vi "Magnet device cluster to String.vi"(11 "Magnet PSU":T1={"Nickname"="", "Bipolar Output"="", "Out Config"="SERS", "Current Limit"=0.0, "AtoB"=0.0, "Inductance"=0.0, "Switch Present"="", "Swh Htr Current"=0.0, "SW VLIM"=0.0, "Ignore Voltage Transient"="", "V Trans Time"=0.0, "Magnet PSU Signals"={"Target Current"=0.0, "Target Field"=0.0, "Target Current Rate"=0.0, "Target Field Rate"=0.0, "Switch Heater Status"="", "Set Switch Heater"="", "PSU Act Stat"="HOLD"}} {"Magnet PSU Signals"."Target Field Rate" min=0.0 max=50.0 step=0.01 format="%#.2f"; "Magnet PSU Signals"."Target Current Rate" min=0.0 max=1200.0 step=0.01 format="%#.2f"; "Magnet PSU Signals"."Target Field" min=-360.0 max=360.0 step=0.01 format="%#.2f"; "Magnet PSU Signals"."Target Current" min=-360.0 max=360.0 step=0.01 format="%#.2f"; "V Trans Time" min=0.0 max=120.0 step=0.01 format="%#.2f"; "SW VLIM" min=0.0 max=12.49 step=0.01 format="%#.2f"; "Swh Htr Current" min=0.0 max=125.0 step=0.01 format="%#.2f"; "Inductance" min=1.0 max=500.0 step=0.01 format="%#.2f"; "AtoB" min=1.0 max=30.0 step=0.01 format="%#.2f"; "Current Limit" min=0.0 max=360.0 step=0.01 format="%#.2f"}) -> (3 "Data to send":string=":NICK:Z-PSU:BIPL:1:OCNF:SERS:SWPR:0:VTRN:1:CLIM:45.00:ATOB:15.00:IND:12.00:SHTC:34.00:VLIM:12.49:VTRT:4.00:SIG:CSET:10.0:FSET:23.0:RCST:4.0:RFST:5.0:SWHT:ON:SWHN:OFF:ACTN:RTOS:SIG")   [LabVIEW 2013, in "Mercury iXX.lvlib" / "Magnet.lvlib"]
uses:
  <instrlib>/Mercury iXX/Public/Libraries/Magnet.lvlib
  <instrlib>/Mercury iXX/Public/Libraries/Magnet/Controls/Device (Set).ctl
  <instrlib>/Mercury iXX/Public/Libraries/Magnet/Controls/Output Configuration.ctl
  <instrlib>/Mercury iXX/Public/Libraries/Magnet/Controls/Signals (Set).ctl
  <instrlib>/Mercury iXX/Public/Libraries/Magnet/Controls/Switch Heater.ctl
  <instrlib>/Mercury iXX/Public/Libraries/Magnet/Controls/PSU Actions.ctl
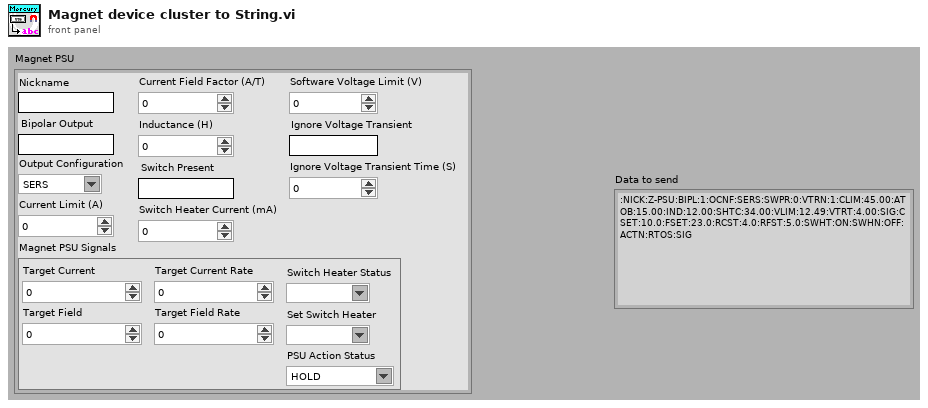
[diagram p1: front panel]
types:
  T1 = typedef "Mercury iXX.lvlib/Magnet.lvlib/Device (Set).ctl" = cluster{"Nickname":string, "Bipolar Output":string, "Out Config":T2, "Current Limit":dbl, "AtoB":dbl, "Inductance":dbl, "Switch Present":string, "Swh Htr Current":dbl, "SW VLIM":dbl, "Ignore Voltage Transient":string, "V Trans Time":dbl, "Magnet PSU Signals":T3}
  T2 = typedef "Mercury iXX.lvlib/Magnet.lvlib/Output Configuration.ctl" = string
  T3 = typedef "Mercury iXX.lvlib/Magnet.lvlib/Signals (Set).ctl" = cluster{"Target Current":dbl, "Target Field":dbl, "Target Current Rate":dbl, "Target Field Rate":dbl, "Switch Heater Status":T4, "Set Switch Heater":T4, "PSU Act Stat":T5}
  T4 = typedef "Mercury iXX.lvlib/Magnet.lvlib/Switch Heater.ctl" = string
  T5 = typedef "Mercury iXX.lvlib/Magnet.lvlib/PSU Actions.ctl" = string
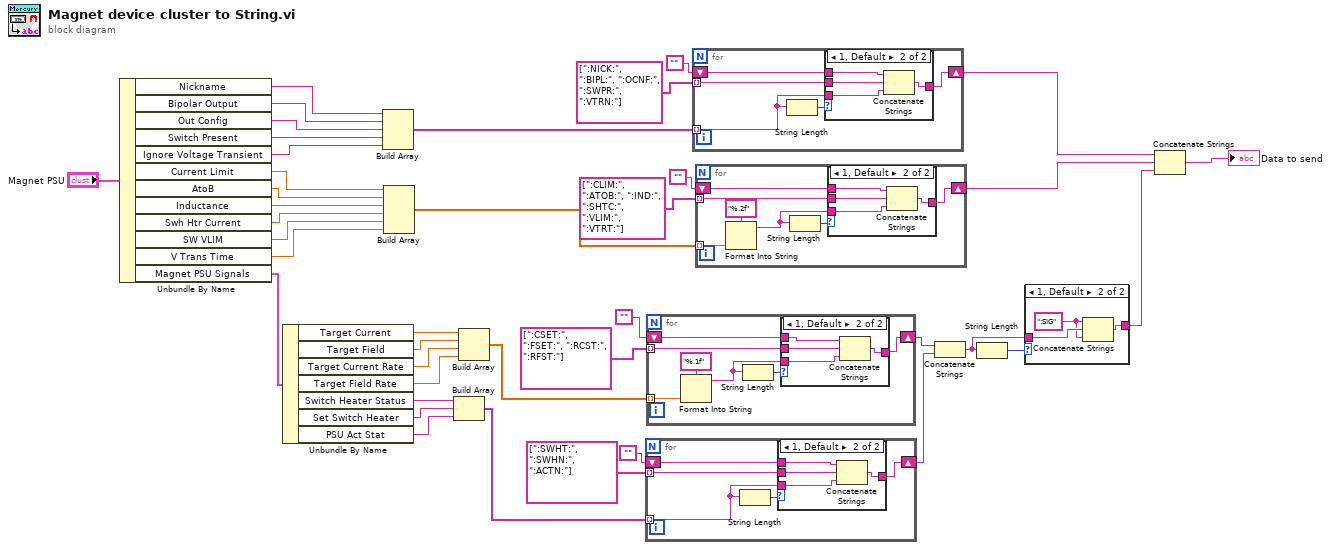
[diagram p0: block diagram]
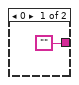
[diagram p4: hidden frame]
diagram:
  n1 = Unbundle By Name("Magnet PSU") -> ("Nickname"=w31:string, "Bipolar Output"=w32:string, "Out Config"=w39:T2, "Switch Present"=w23:string, "Ignore Voltage Transient"=w22:string, "Current Limit"=w21:dbl, "AtoB"=w20:dbl, "Inductance"=w19:dbl, "Swh Htr Current"=w18:dbl, "SW VLIM"=w16:dbl, "V Trans Time"=w17:dbl, "Magnet PSU Signals"=w15:T3)
  n2 = Unbundle By Name(w15) -> ("Target Current"=w14:dbl, "Target Field"=w13:dbl, "Target Current Rate"=w12:dbl, "Target Field Rate"=w11:dbl, "Switch Heater Status"=w10:T4, "Set Switch Heater"=w9:T4, "PSU Act Stat"=w8:T5)
  n3 = Build Array(w31, w32, w39, w23, w22) -> (w30:T2[])
  n4 = Build Array(w21, w20, w19, w18, w16, w17) -> (w26:dbl[])
  n5 = Build Array(w10, w9, w8) -> (w5:T5[])
  n6 = Build Array(w14, w13, w12, w11) -> (w7:dbl[])
  n7 = for {
    tunnel: w5 -> [w41] mode=indexing
    tunnel: string[] [":SWHT:", ":SWHN:", ":ACTN:"] ("Excitation") -> [w44] mode=indexing
    shift-right: [w43] -> w1
    shift-left: "" -> [w42]
    n8 = String Length(string=w41) -> (length=w45:i32)
    n9 = case shown="1, Default" w45 {
      tunnel: w41 -> [_ w49]
      tunnel: [w46 w50] -> w43
      tunnel: w44 -> [_ w48]
      tunnel: w42 -> [w46 w47]
      frame 0 {
      }
      frame 1, Default {
        n10 = Concatenate Strings(w47, w48, w49) -> (w50:string)
      }
    }
  }
  n11 = for {
    tunnel: w7 -> [w51] mode=indexing
    tunnel: string[] [":CSET:", ":FSET:", ":RCST:", ":RFST:"] ("Excitation") -> [w56] mode=indexing
    shift-right: [w54] -> w3
    shift-left: "" -> [w55]
    n12 = Format Into String(format string="%.1f", w51) -> (resulting string=w52:string)  [unwired: 2 in, 1 out]
    n13 = String Length(string=w52) -> (length=w57:i32)
    n14 = case shown="1, Default" w57 {
      tunnel: w52 -> [_ w61]
      tunnel: [w58 w62] -> w54
      tunnel: w56 -> [_ w60]
      tunnel: w55 -> [w58 w59]
      frame 0 {
      }
      frame 1, Default {
        n15 = Concatenate Strings(w59, w60, w61) -> (w62:string)
      }
    }
  }
  n16 = for {
    tunnel: w30 -> [w63] mode=indexing
    tunnel: string[] [":NICK:", ":BIPL:", ":OCNF:", ":SWPR:", ":VTRN:"] ("Excitation") -> [w66] mode=indexing
    shift-right: [w65] -> w33
    shift-left: "" -> [w64]
    n17 = String Length(string=w63) -> (length=w67:i32)
    n18 = case shown="1, Default" w67 {
      tunnel: w63 -> [_ w71]
      tunnel: [w68 w72] -> w65
      tunnel: w66 -> [_ w70]
      tunnel: w64 -> [w68 w69]
      frame 0 {
      }
      frame 1, Default {
        n19 = Concatenate Strings(w69, w70, w71) -> (w72:string)
      }
    }
  }
  n20 = for {
    tunnel: w26 -> [w75] mode=indexing
    tunnel: string[] [":CLIM:", ":ATOB:", ":IND:", ":SHTC:", ":VLIM:", ":VTRT:"] ("Excitation") -> [w78] mode=indexing
    shift-right: [w77] -> w24
    shift-left: "" -> [w76]
    n21 = Format Into String(format string="%.2f", w75) -> (resulting string=w74:string)  [unwired: 2 in, 1 out]
    n22 = String Length(string=w74) -> (length=w79:i32)
    n23 = case shown="1, Default" w79 {
      tunnel: w74 -> [_ w83]
      tunnel: [w80 w84] -> w77
      tunnel: w78 -> [_ w82]
      tunnel: w76 -> [w80 w81]
      frame 0 {
      }
      frame 1, Default {
        n24 = Concatenate Strings(w81, w82, w83) -> (w84:string)
      }
    }
  }
  n25 = Concatenate Strings(w3, w1) -> (w2:string)
  n26 = String Length(string=w2) -> (length=w29:i32)
  n27 = case shown="1, Default" w29 {
    tunnel: ["" w88] -> w25
    tunnel: w2 -> [_ w87]
    frame 0 {
    }
    frame 1, Default {
      w86 = ":SIG" ("string")
      n28 = Concatenate Strings(w86, w87, w86) -> (w88:string)
    }
  }
  n29 = Concatenate Strings(w33, w24, w25) -> (→"Data to send":string)
